vi "Test Correct Data is Sent When Measuring DC Voltage.vi"(8 "error in (no error)":errorcluster, 11 "Test Case In":refnum<class "Low Level PSU Test.lvclass">) -> (0 "error out":errorcluster, 3 "Test Case Out":refnum<class "Low Level PSU Test.lvclass">)   [LabVIEW 2020, in "Low Level PSU With Tests.lvlib" / "Low Level PSU Test.lvclass"]
uses:
  Low Level PSU Test.lvclass
  Low Level PSU Test.lvclass/Low Level PSU Test.ctl
  01074fa8-ee8a-411d-bc8b-fc92c4f90959.vi
  Mock Instrument Interface/Mock Instrument.lvclass
  Low Level PSU/Low Level PSU.lvclass
  C:/Git/astemes-gdevcon-2022/PSU Demo/Low Level PSU With Tests/Mock Instrument Interface/Mock Instrument.lvclass
  C:/Git/astemes-gdevcon-2022/PSU Demo/Low Level PSU With Tests/Instrument Interface/Instrument.lvclass
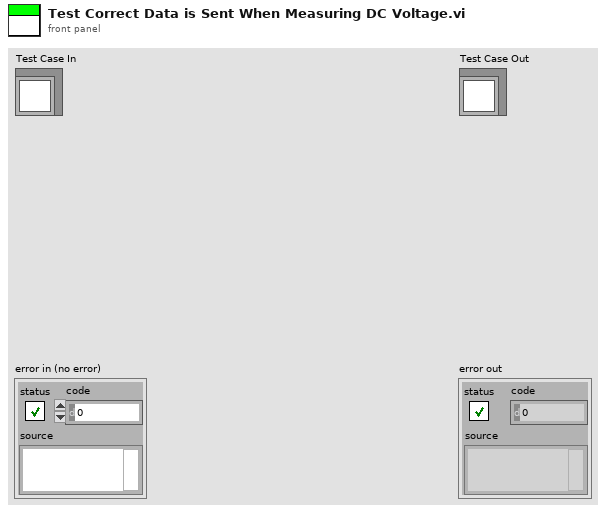
[diagram p1: front panel]
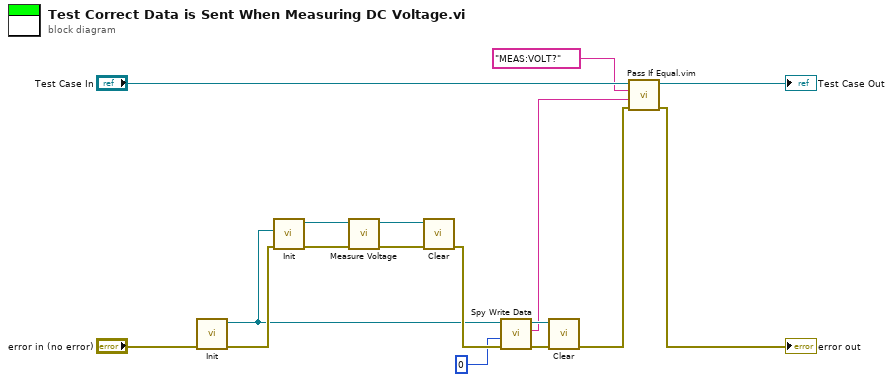
[diagram p0: block diagram]
diagram:
  n1 = call "Init.vi"("error in (no error)"="error in (no error)") -> ("error out"=w12:errorcluster, "Mock Instrument Interface Out"=w5:refnum<class "Mock Instrument.lvclass">)  [unwired: 9 in]
  n2 = call "Init.vi"("error in (no error)"=w12, "Instrument Interface"=w5) -> ("error out"=w13:errorcluster, "Low Level PSU Out"=w14:refnum<class "Low Level PSU.lvclass">)  [unwired: 8 in]
  n3 = call "Measure Voltage.vi"("error in (no error)"=w13, "Low Level PSU In"=w14) -> ("error out"=w9:errorcluster, "Low Level PSU Out"=w10:refnum<class "Low Level PSU.lvclass">)  [unwired: 7 in, 1 out]
  n4 = call "Clear.vi"("error in (no error)"=w9, "Low Level PSU In"=w10) -> ("error out"=w6:errorcluster)  [unwired: 8 in, 1 out]
  n5 = call "Spy Write Data.vi"("error in (no error)"=w6, "timeout in ms (-1)"=0, "Mock Instrument Interface in"=w5) -> ("error out"=w7:errorcluster, "Data"=w3:string, "Mock Instrument Interface out"=w8:refnum<class "Mock Instrument.lvclass">)  [unwired: 5 in, 1 out]
  n6 = call "Clear.vi"("error in (no error)"=w7, "Mock Instrument Interface In"=w8) -> ("error out"=w1:errorcluster)  [unwired: 8 in, 1 out]
  n7 = call "Pass If Equal.vim"("error in (no error)"=w1, "Actual"=w3, "Expected"="MEAS:VOLT?" ("Data"), "LUnit Test Case In"="Test Case In") -> ("error out"=→"error out":errorcluster, "LUnit Test Case Out"=→"Test Case Out":refnum<class "Low Level PSU Test.lvclass">)  [unwired: 6 in]
